vi "DCS_Waveform_Processing.vi"(6 "DAQ Sample Window (2000)":i32=2000, 8 "Rank (20)":i32=20, 9 "DAQ bit size (16)":u16=16, 10 "Max Voltage Amplitude (2.5 V)":dbl=2.5, 11 "Raw Data":dbl[][](array[numeric])) -> (0 "Second Plane Max Value Index":i32, 1 "Voltage Data":dbl[][](array[numeric]), 2 "Trimmed Waveform":ext[][](array[numeric]), 3 "Good Signal":bool, 4 "First Plane Max Value Index":i32)   [LabVIEW 2015]
doc: "Takes raw data from DCS DAQ, converts to voltage, checks for good signal, and trims waveform around wire plane peak values."
panel:
  out "First Plane":ext[][](graph)
  out "Second Plane":ext[][](graph)
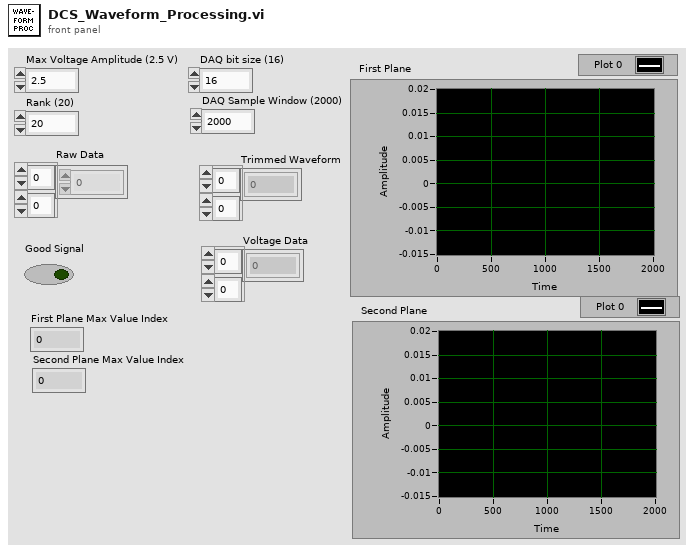
[diagram p1: front panel]
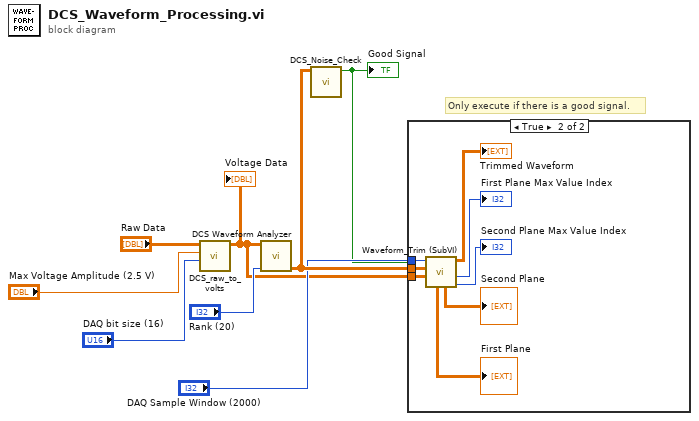
[diagram p0: block diagram]
diagram:
  # "Only execute if there is a good signal."
  n1 = call "DCS_raw_to_volts.vi"("DAQ bit size (16)"="DAQ bit size (16)", "Max Voltage Amplitude (2.5 V)"="Max Voltage Amplitude (2.5 V)", "Raw Data"="Raw Data") -> ("Voltage Data"=w2:dbl[][])  [unwired: 8 in]
  "Voltage Data" <- w2
  n2 = call "DCS Waveform Analyzer.vi"("Rank"="Rank (20)", "8 DCS Waveforms"=w2) -> ("Filtered Signals"=w4:dbl[][])  [unwired: 8 in, 1 out]
  n3 = call "DCS_Noise_Check.vi"("8 DCS Waveforms"=w4) -> ("Boolean"=w1:bool)  [unwired: 10 in]
  "Good Signal" <- w1
  n4 = case shown="True" w1 {
    tunnel: w4 -> [_ w16]
    tunnel: "DAQ Sample Window (2000)" -> [_ w15]
    tunnel: w2 -> [_ w14]
    frame False {
    }
    frame True {
      n5 = call "Waveform_Trim (SubVI).vi"("Raw Waveform"=w14, "Filtered Waveform"=w16, "DAQ Sample Window"=w15) -> ("Second Plane Max Value Index"=→"Second Plane Max Value Index":i32, "First Plane Max Value Index"=→"First Plane Max Value Index":i32, "Trimmed Waveform"=→"Trimmed Waveform":ext[][], "Second Plane"=→"Second Plane":ext[][], "First Plane"=→"First Plane":ext[][])  [unwired: 4 in]
    }
  }
